vi "Run_Pre Core.vi"(0 "For Loop in":refnum<class "Structure If Else.lvclass">, 11 "error in (no error)":errorcluster) -> (4 "For Loop out":refnum<class "Structure If Else.lvclass">, 6 "Go to Run Pre Core?":bool, 15 "error out":errorcluster)   [LabVIEW 2019, in "Structure If Else.lvclass"]
uses:
  Structure If Else.lvclass
  Structure If Else.lvclass/Structure If Else.ctl
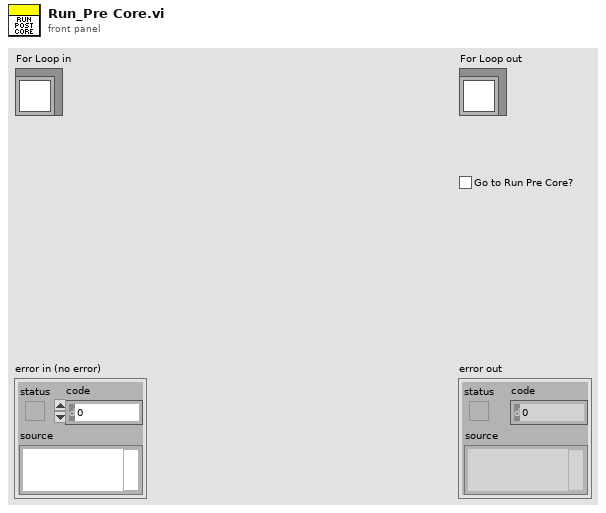
[diagram p1: front panel]
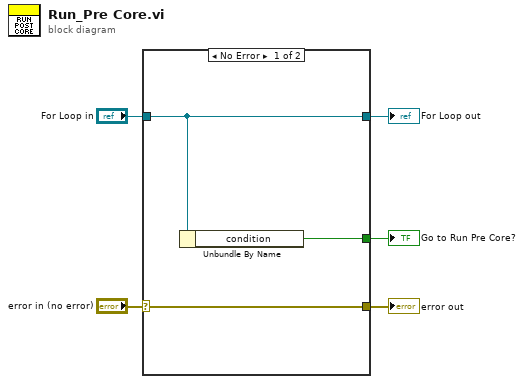
[diagram p0: block diagram]
diagram:
  n1 = case shown="No Error" "error in (no error)" {
    selector: "error in (no error)" -> [w8 w10]
    tunnel: "For Loop in" -> [w7 w9]
    tunnel: [w8 w10] -> w4
    tunnel: [w7 w9] -> w2
    tunnel: [w6 _] -> w1
    frame No Error {
      n2 = Unbundle By Name(w7) -> ("condition"=w6:bool)
    }
    frame Error {
    }
  }
  "error out" <- w4
  "For Loop out" <- w2
  "Go to Run Pre Core?" <- w1
